vi "Download Bitfile.vi"(8 "error in (no error)":errorcluster, 11 "starter kit FPGA host in":refnum<class "NI_Robotics_Starter Kit Host_FPGA.lvclass">) -> (0 "error out":errorcluster, 3 "starter kit FPGA host out":refnum<class "NI_Robotics_Starter Kit Host_FPGA.lvclass">)   [LabVIEW 2017, in "NI_Robotics_Starter Kit Host_FPGA.lvclass"]
uses:
  <vilib>/robotics/Starter Kit/FPGA Host Interface/NI_Robotics_Starter Kit Host_FPGA.lvclass
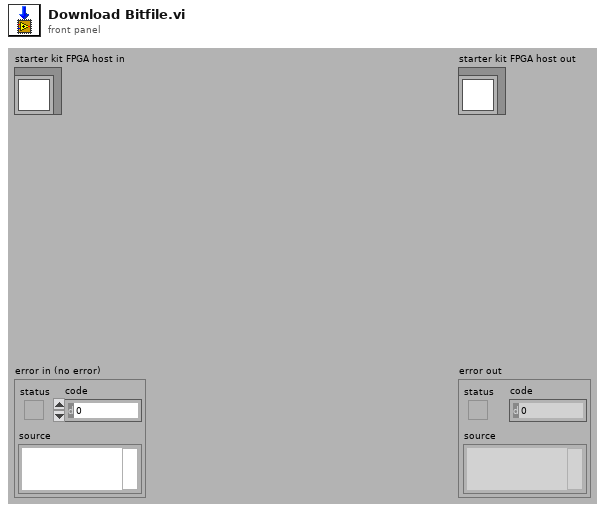
[diagram p1: front panel]
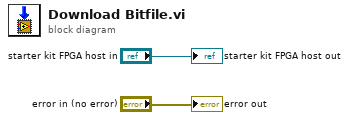
[diagram p0: block diagram]
diagram:
  "error out" <- "error in (no error)"
  "starter kit FPGA host out" <- "starter kit FPGA host in"
